vi "MotorSpeedMeng.vi"(8 "Motor settings (X,Y)":cluster{"Vmax (mm/s)":sgl, "Acc (mm/s/s)":sgl}={"Vmax (mm/s)"=0.1, "Acc (mm/s/s)"=0.5}, 9 "Enum":enum16{"Int", "Set"}(ring), 10 "error in (no error)":errorcluster, 11 "Automation Refnum in":refnum<k7>) -> (2 "error out":errorcluster, 3 "Automation Refnum out":refnum<k7>)   [LabVIEW 2014]
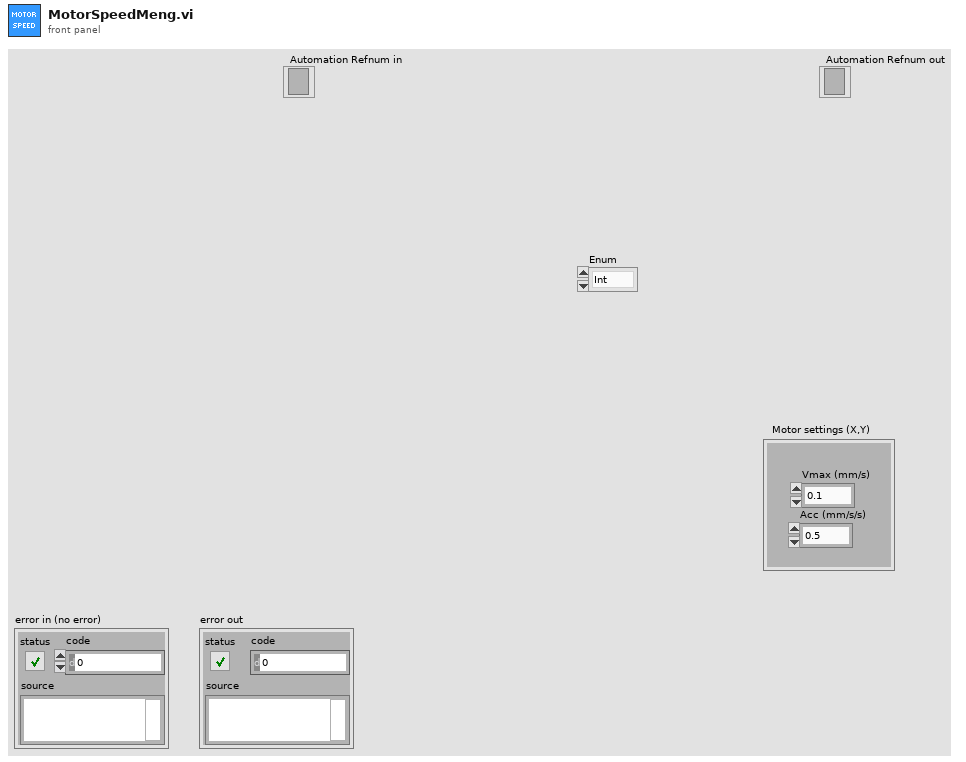
[diagram p1: front panel]
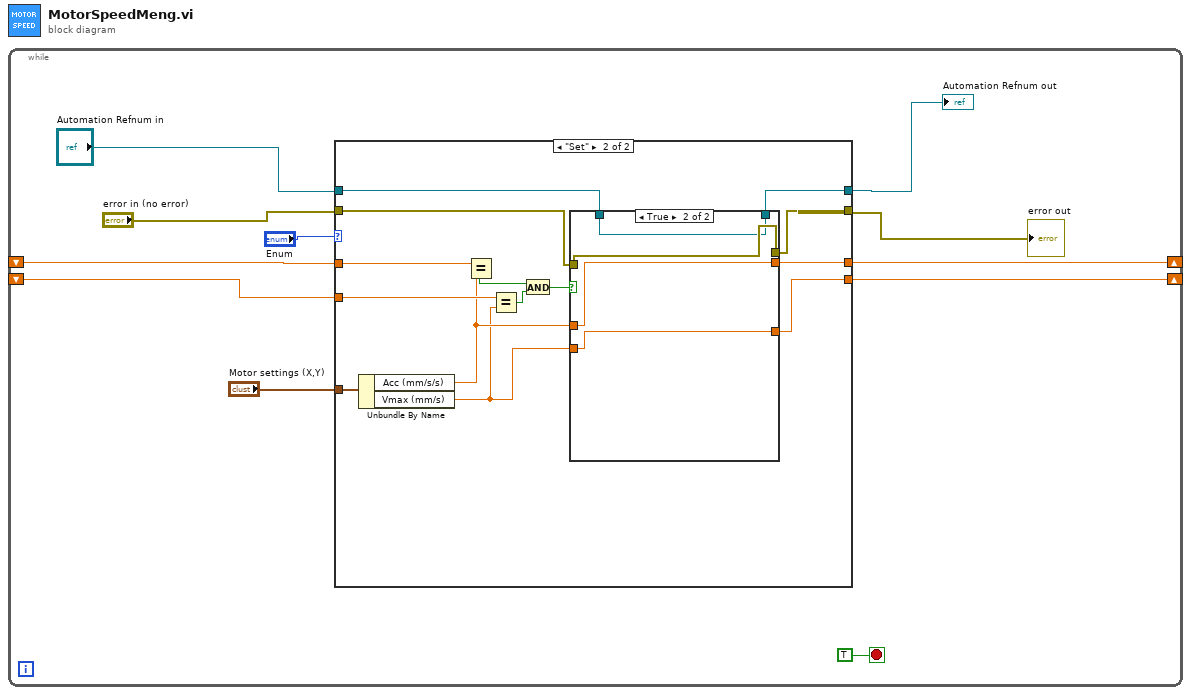
[diagram p0: block diagram]
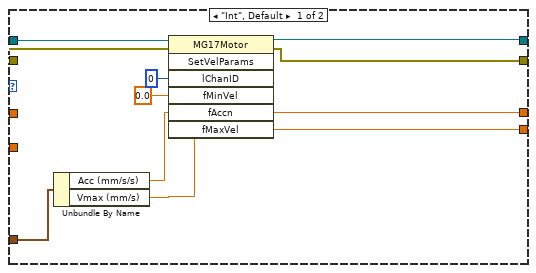
[diagram p2: hidden frame]
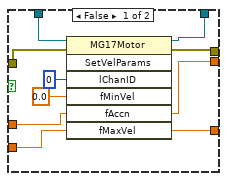
[diagram p3: hidden frame]
diagram:
  n1 = while {
    shift-right: [w8] -> _
    shift-left: _ -> [w6]
    shift-right: [w7] -> _
    shift-left: _ -> [w5]
    stop <- TRUE stop-if-true
    n2 = case shown="\"Set\"" "Enum" {
      tunnel: "Automation Refnum in" -> [w22 w27]
      tunnel: [w20 w28] -> w1
      tunnel: [w19 w29] -> w2
      tunnel: "error in (no error)" -> [w21 w30]
      tunnel: "Motor settings (X,Y)" -> [w14 w36]
      tunnel: [w13 w24] -> w8
      tunnel: [w12 w23] -> w7
      tunnel: w6 -> [_ w35]
      tunnel: w5 -> [_ w34]
      frame "Int", Default {
        n3 = Unbundle By Name(w14) -> ("Acc (mm/s/s)"=w16:sgl, "Vmax (mm/s)"=w15:sgl)
        n4 = invoke class="MG17Motor" method="SetVelParams"(reference=w22, error in=w21, "lChanID"=0, "fMinVel"=sgl 0.0, "fAccn"=w16, "fMaxVel"=w15) -> (reference out=w20:refnum<k7>, error out=w19:errorcluster, "fAccn"=w13:sgl, "fMaxVel"=w12:sgl)  [unwired: 1 in, 3 out]
      }
      frame "Set" {
        n5 = Unbundle By Name(w36) -> ("Acc (mm/s/s)"=w26:sgl, "Vmax (mm/s)"=w25:sgl)
        n6 = Equal?(x=w35, y=w26) -> (x = y?=w33:bool)
        n7 = Equal?(x=w34, y=w25) -> (x = y?=w32:bool)
        n8 = And(x=w33, y=w32) -> (x .and. y?=w31:bool)
        n9 = case shown="True" w31 {
          tunnel: w30 -> [w46 w50]
          tunnel: w27 -> [w45 w49]
          tunnel: [w44 w50] -> w29
          tunnel: [w41 w49] -> w28
          tunnel: w26 -> [w40 w48]
          tunnel: w25 -> [w39 w47]
          tunnel: [w38 w48] -> w24
          tunnel: [w37 w47] -> w23
          frame False {
            n10 = invoke class="MG17Motor" method="SetVelParams"(reference=w45, error in=w46, "lChanID"=0, "fMinVel"=sgl 0.0, "fAccn"=w40, "fMaxVel"=w39) -> (reference out=w41:refnum<k7>, error out=w44:errorcluster, "fAccn"=w38:sgl, "fMaxVel"=w37:sgl)  [unwired: 1 in, 3 out]
          }
          frame True {
          }
        }
      }
    }
    "Automation Refnum out" <- w1
    "error out" <- w2
  }
